vi "SimulationsLIA-Simulator.vi"() -> ()   [LabVIEW 2018]
uses:
  <vilib>/addons/Digital Filter Design/_Objects.llb/DFD Multirate Filter Specification (Design).ctl
  <vilib>/addons/Digital Filter Design/_Objects.llb/DFD Filter Ripple Specification (Design).ctl
  <vilib>/Analysis/4window.llb/windowTd.ctl
  <vilib>/addons/Digital Filter Design/Design.llb/DFD MRate Filter Design (Integer).vi
  <vilib>/addons/Digital Filter Design/Multirate.llb/DFD MRate Filtering (Array).vi
  <vilib>/measure/maspectr.llb/FFT Power Spectrum and PSD for 1 Chan (CDB).vi
  <vilib>/measure/maspectr.llb/FFT Power Spectrum and PSD for 1 Chan.vi
  <vilib>/measure/NI_MAPro.lvlib
  <vilib>/Analysis/NI_AALPro.lvlib
  <vilib>/addons/Digital Filter Design/NI_DigFilterLicensed.lvlib
  <vilib>/Analysis/NI_AALBase.lvlib
  <vilib>/addons/Digital Filter Design/Analysis.llb/DFD Plot Freq Response (Linear-Spaced).vi
panel:
  in  "Iterations":i32=10
  out "FFT Gain":dbl
  out "Audio Depth":dbl format="%#_p"
  in  "Resolution":dbl=19.0 format="%#_13g"
  in  "Sampling Rate":dbl=1.0 format="%#_p"
  in  "Number Samples":i32=10000
  out "Error Out":errorcluster
  in  "Error In":errorcluster
  in  "Stop":bool
  in  "Tab Control 3":enum32{"Signal", "Noise", "Decimated"}(tab)
  out "Noise vrms":dbl
  out "Noise (W|50ohms)":dbl
  out "k":dbl
  out "standard deviation":dbl format="%0.2p"
  out "mean":dbl format="%0.2p"
  in  "Tab Control 2":T1(tab)
  out "Waveform Graph 1":dbl[][](graph)
  out "Waveform Graph 3":cluster{"f0":dbl, "df":dbl, "magnitude":dbl[]}(graph)
  out "Waveform Graph 8":dbl[][](graph)
  out "Waveform Graph 7":cluster{"f0":dbl, "df":dbl, "magnitude":dbl[]}(graph)
  out "Waveform Graph 10":dbl[](graph)
  out "Waveform Graph 9":cluster{"f0":dbl, "df":dbl, "magnitude":dbl[]}(graph)
  out "Waveform Graph 12":dbl[](graph)
  out "Waveform Graph 11":cluster{"f0":dbl, "df":dbl, "magnitude":dbl[]}(graph)
  out "Waveform Graph 14":dbl[][](graph)
  out "Waveform Graph 13":cluster{"f0":dbl, "df":dbl, "magnitude":dbl[]}(graph)
  out "Waveform Graph 16":dbl[](graph)
  out "Waveform Graph 15":cluster{"f0":dbl, "df":dbl, "magnitude":dbl[]}(graph)
  in  "Tab Control 1":T2(tab)
  in  "Oscillator Frequency":dbl=-0.1 format="%#_p"
  in  "Oscillator Magnitude":dbl=1.0 format="%#_13g"
  in  "Signal Frequency":dbl=0.1 format="%#_p"
  in  "Signal Offset":cdb format="%#_13g"
  in  "Singal Amplitude":dbl=1.0 format="%#_13g"
  in  "Desired SNR (dB)":dbl format="%#_p"
  in  "freq specs [Hz]":T3={"fpass"=0.001, "fstop"=0.002}
  in  "ripple specs":T4={"passband"=0.1, "stopband"=70.0, "dB/linear? (T: dB)"=TRUE}
  in  "Decimation":i32=100
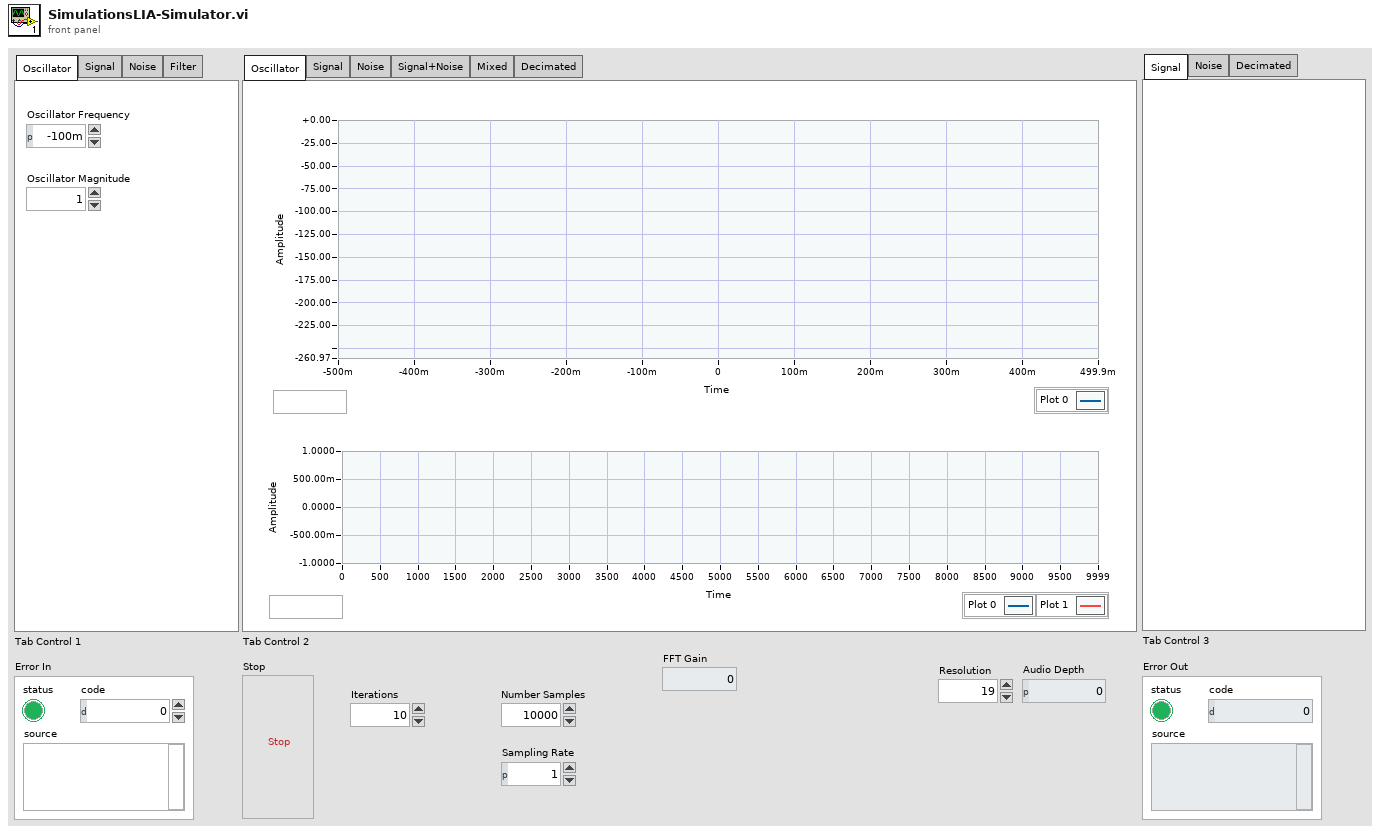
[diagram p1: front panel]
types:
  T1 = enum32{"Oscillator", "Signal", "Noise", "Signal+Noise", "Mixed", "Decimated"}
  T2 = enum32{"Oscillator", "Signal", "Noise", "Filter"}
  T3 = typedef "NI_DigFilterLicensed.lvlib/DFD Multirate Filter Specification (Design).ctl" = cluster{"fpass":dbl, "fstop":dbl}
  T4 = typedef "NI_DigFilterLicensed.lvlib/DFD Filter Ripple Specification (Design).ctl" = cluster{"passband":dbl, "stopband":dbl, "dB/linear? (T: dB)":bool}
  T5 = typedef "NI_DigFilterLicensed.lvlib/DFD Multirate Filter Obj.ctl" = cluster{"mMRate_Structure":enum16{"CIC", "FIR", "IIR", "Lattice"}, "mMRate_Mode":T6, "mMRate_Factor":i32, "mMRate_FIRParams":cluster{"mMRate_FIR_H":dbl[], "mMRate_FIR_IsNyquist?":bool, "mMRate_FIR_IsSymmetric?":bool}, "mMRate_CICParams":cluster{"mMRate_CIC_#Stage":i32, "mMRate_CIC_Lag":i32, "mMRate_CIC_Type":enum16{"Lowpass", "Highpass"}}, "mMRate_Order":i32, "mMRate_Version":string, "mMRate_Comments":string, "mMRate_RationalFactor":cluster{"mMRate_L":i32, "mMRate_M":i32}, "mMRate_Fs":dbl, "mMRate_Quantized?":bool, "mMRate_QFilterGain":dbl, "mMRate_CoefWl":i16, "mMRate_Scaling":cluster{"mMRate_ScaleByPowerOf2?":bool, "mMRate_ScaleType":T7}, "mMRate_InputWl":i16, "mMRate_OutputWl":i16, "mMRate_OutputMode":T8, "mMRate_MultMode":T9, "mMRate_BitPruning":bool, "mMRate_GainWl":i16, "mMRate_OutputFwl":i16, "mMRate_SumIwl":i16, "mMRate_InputIwl ":i16, "mMRate_SumWl":i16, "mMRate_CoefIwl":i16}
  T6 = typedef "NI_DigFilterLicensed.lvlib/DFD Multirate Mode.ctl" = i16
  T7 = typedef "NI_DigFilterLicensed.lvlib/DFD Coef Norm Type.ctl" = enum16{"No Norm", "Time Domain 1-Norm", "Time Domain 2-Norm", "Time Domain Inf-Norm"}
  T8 = typedef "NI_DigFilterLicensed.lvlib/DFD Round-off Mode.ctl" = enum16{"Nearest", "Truncation"}
  T9 = typedef "NI_DigFilterLicensed.lvlib/DFD FXP MRate Multiply Mode.ctl" = enum16{"Truncated", "Full"}
  T10 = cluster{"averaging mode":enum16{"No averaging", "Vector averaging", "RMS averaging", "Peak hold"}, "weighting mode":enum16{"Linear", "Exponential"}, "number of averages":u32}
  T11 = typedef "NI_AALPro.lvlib/windowTd.ctl" = u32
  T12 = typedef "NI_DigFilterLicensed.lvlib/DFD Filter Obj.ctl" = cluster{"mSRate_Fs":dbl, "mSRate_Version":string, "mSRate_Comments":string, "mSRate_OrgCoef":T13, "mSRate_CurCoef":T13, "mSRate_Quantized?":bool, "mSRate_QCoef":T13, "mSRate_QSettings":T15[], "mSRate_Order":i32, "mSRate_Scaling":cluster{"mSRate_ScaleByPowerOf2?":bool, "mSRate_ScaleType":T7}}
  T13 = typedef "NI_DigFilterLicensed.lvlib/DFD Filter Coef.ctl" = cluster{"type":T14, "gain":dbl, "coef a (k)":dbl[], "coef b (v)":dbl[]}
  T14 = typedef "NI_DigFilterLicensed.lvlib/DFD Filter Structure Type Selector.ctl" = enum16{"Undefined", "FIR Direct Form", "FIR Direct Form Transposed", "FIR Symmetric", "FIR Antisymmetric", "IIR Direct Form I", "IIR Direct Form I Transposed", "IIR Direct Form II", "IIR Direct Form II Transposed", "IIR Cascaded Second Order Sections Form I", "IIR Cascaded Second Order Sections Form I Transposed", "IIR Cascaded Second Order Sections Form II", "IIR Cascaded Second Order Sections Form II Transposed", "Lattice Allpass (basic sections)", "Lattice Allpass (one multiplier sections)", "Lattice Allpass (normalized sections)", "Lattice AR (basic sections)", "Lattice AR (one multiplier sections)", "Lattice AR (normalized sections)", "Lattice MA (minimum phase)", "Lattice MA (maximum phase)", "Lattice ARMA (basic sections)", "Lattice ARMA (one multiplier sections)", "Lattice ARMA (normalized sections)"}
  T15 = typedef "NI_DigFilterLicensed.lvlib/dfd_Internal Quantization Settings.ctl" = cluster{"source":T16, "wl":i16, "iwl":i16, "overflow mode":enum16{"Saturation", "Wrap"}, "rounding mode":enum16{"Nearest", "Truncation"}, "signed?":bool}
  T16 = typedef "NI_DigFilterLicensed.lvlib/dfd_Internal Quantization Srcs.ctl" = u16
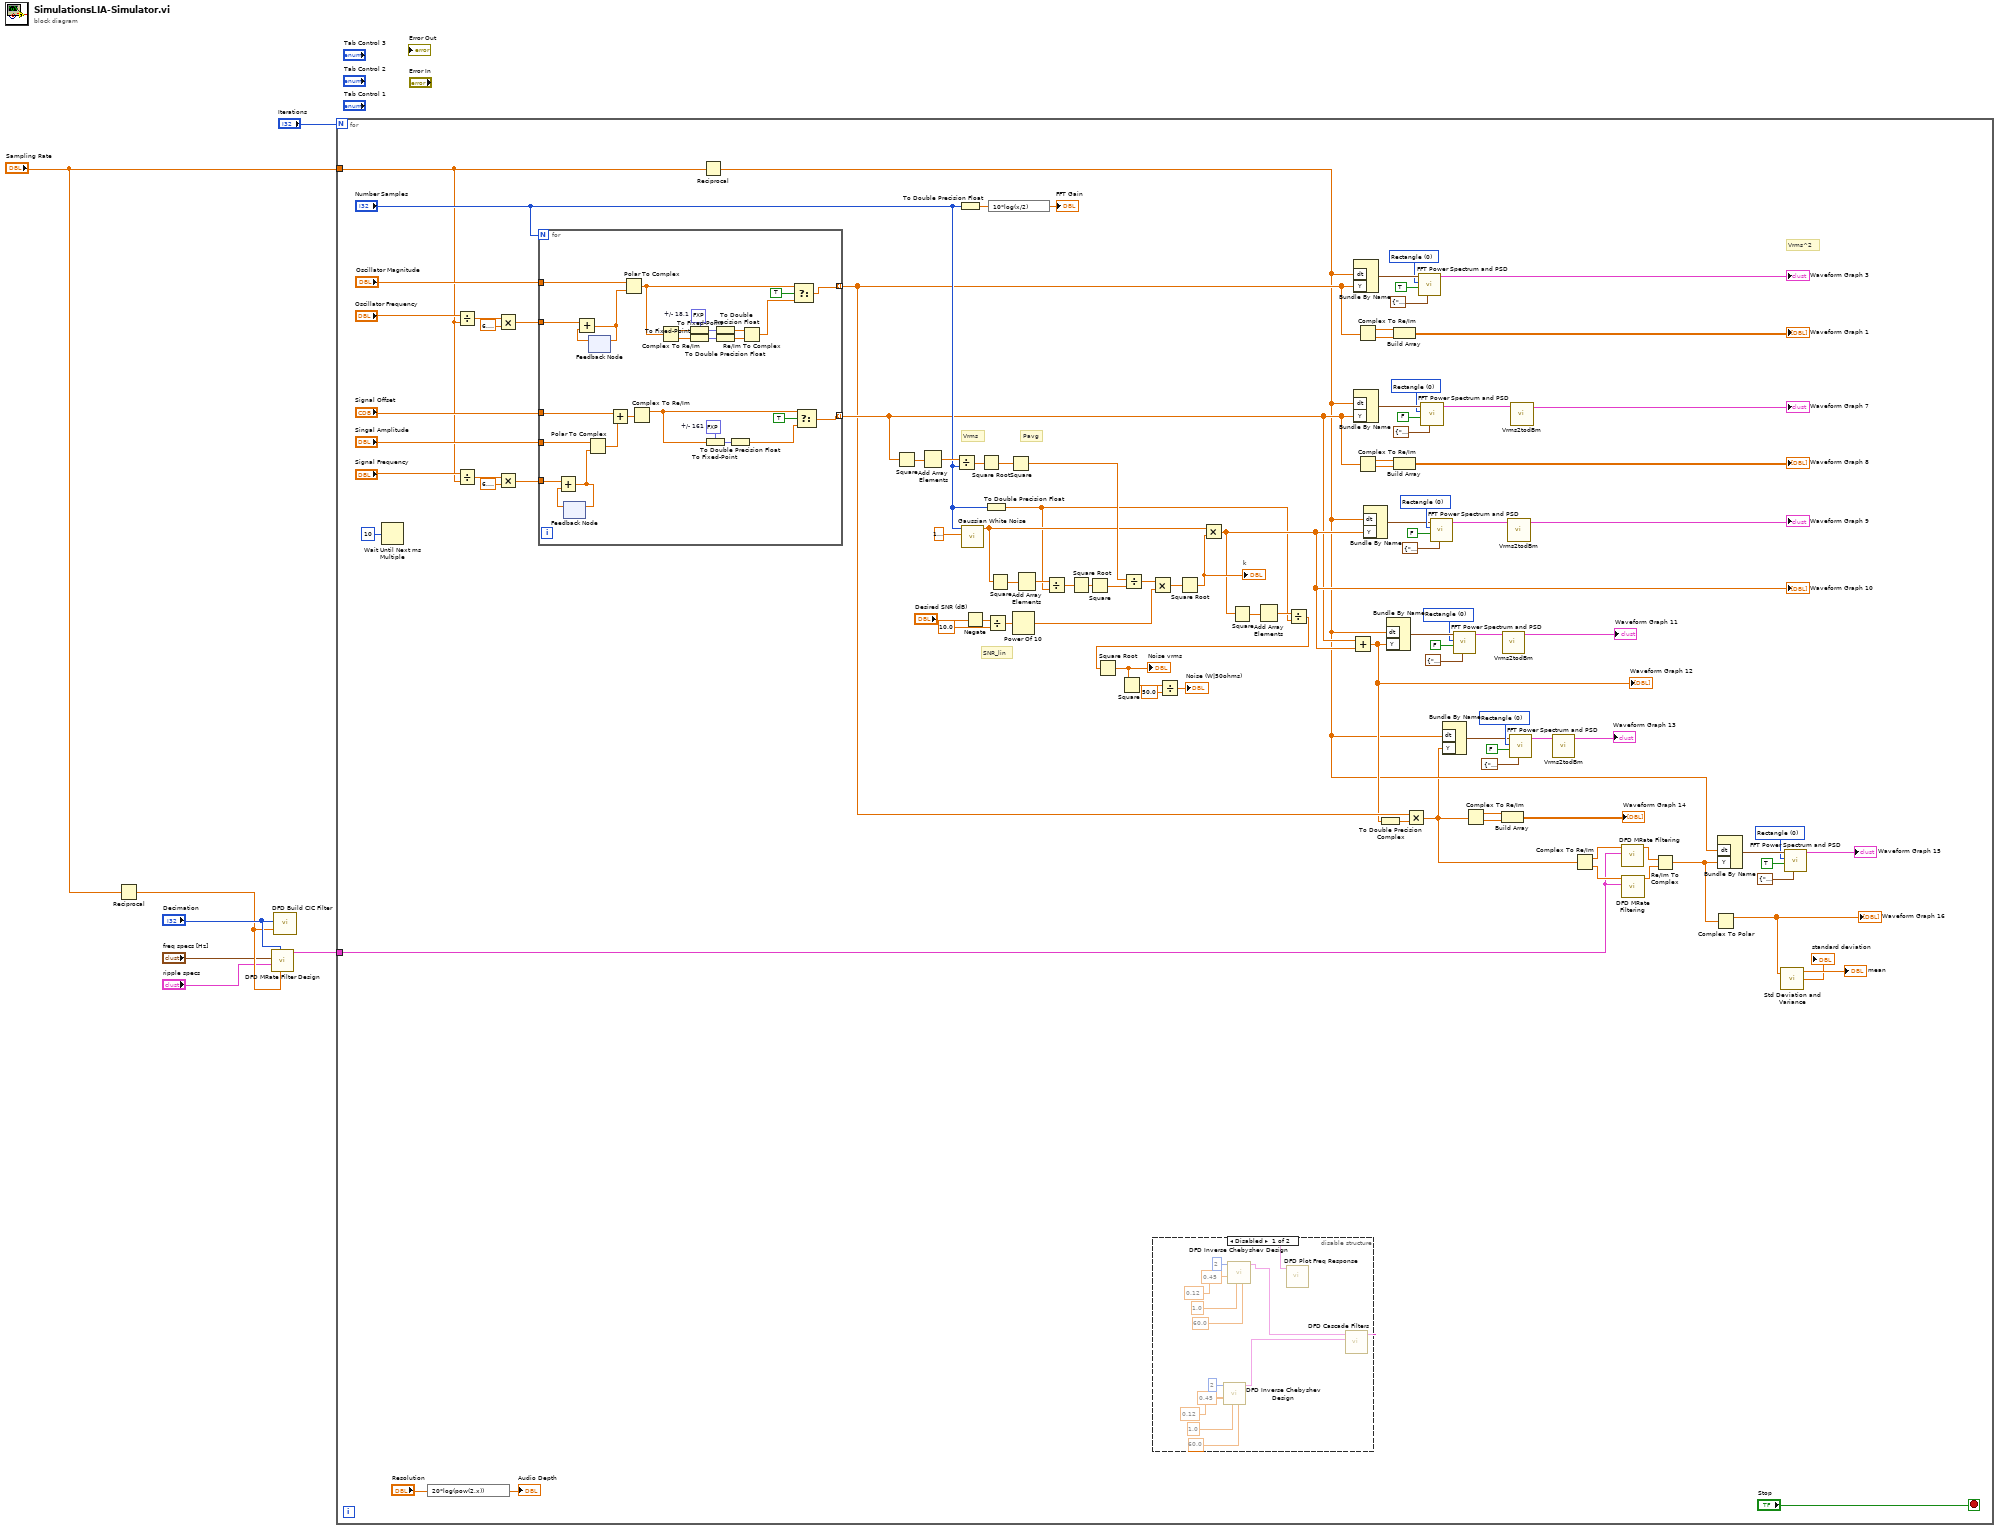
[diagram p0: block diagram]
diagram:
  n1 = Reciprocal(x="Sampling Rate") -> (1/x=w6:dbl)
  n2 = call-poly <vilib>:"DFD MRate Filter Design.vi"("fs in [Hz]"=w6, "factor"="Decimation", "ripple specs"="ripple specs", "freq specs [Hz]"="freq specs [Hz]") -> ("multirate filter out"=w2:T5)  [unwired: 6 in, 1 out]
  n3 = call <vilib>:"DFD Build CIC Filter.vi"("fs in [Hz]"=w6, "factor"="Decimation") -> ()  [unwired: 8 in, 2 out]
  n4 = for {
    N: "Iterations" -> [_]
    tunnel: "Sampling Rate" -> [w13]
    tunnel: w2 -> [w12]
    stop <- "Stop" stop-if-true
    w21 = T11 0 items=["Rectangle"=0, "Hanning"=1, "Hamming"=2, "Blackman-Harris"=3, "Exact Blackman"=4, "Blackman"=5, "Flat Top"=6, "4 Term B-Harris "=7, "7 Term B-Harris"=8, "Low Sidelobe"=9, "Blackman Nuttall"=11, "Triangle"=30, "Bartlett-Hanning"=31, "Bohman"=32, "Parzen"=33, "Welch"=34, "Kaiser"=60, "Dolph-Chebyshev"=61, "Gaussian"=62] ("window")
    w36 = T11 0 items=["Rectangle"=0, "Hanning"=1, "Hamming"=2, "Blackman-Harris"=3, "Exact Blackman"=4, "Blackman"=5, "Flat Top"=6, "4 Term B-Harris "=7, "7 Term B-Harris"=8, "Low Sidelobe"=9, "Blackman Nuttall"=11, "Triangle"=30, "Bartlett-Hanning"=31, "Bohman"=32, "Parzen"=33, "Welch"=34, "Kaiser"=60, "Dolph-Chebyshev"=61, "Gaussian"=62] ("window")
    w47 = T11 0 items=["Rectangle"=0, "Hanning"=1, "Hamming"=2, "Blackman-Harris"=3, "Exact Blackman"=4, "Blackman"=5, "Flat Top"=6, "4 Term B-Harris "=7, "7 Term B-Harris"=8, "Low Sidelobe"=9, "Blackman Nuttall"=11, "Triangle"=30, "Bartlett-Hanning"=31, "Bohman"=32, "Parzen"=33, "Welch"=34, "Kaiser"=60, "Dolph-Chebyshev"=61, "Gaussian"=62] ("window")
    w89 = T11 0 items=["Rectangle"=0, "Hanning"=1, "Hamming"=2, "Blackman-Harris"=3, "Exact Blackman"=4, "Blackman"=5, "Flat Top"=6, "4 Term B-Harris "=7, "7 Term B-Harris"=8, "Low Sidelobe"=9, "Blackman Nuttall"=11, "Triangle"=30, "Bartlett-Hanning"=31, "Bohman"=32, "Parzen"=33, "Welch"=34, "Kaiser"=60, "Dolph-Chebyshev"=61, "Gaussian"=62] ("window")
    w93 = T11 0 items=["Rectangle"=0, "Hanning"=1, "Hamming"=2, "Blackman-Harris"=3, "Exact Blackman"=4, "Blackman"=5, "Flat Top"=6, "4 Term B-Harris "=7, "7 Term B-Harris"=8, "Low Sidelobe"=9, "Blackman Nuttall"=11, "Triangle"=30, "Bartlett-Hanning"=31, "Bohman"=32, "Parzen"=33, "Welch"=34, "Kaiser"=60, "Dolph-Chebyshev"=61, "Gaussian"=62] ("window")
    w101 = T11 0 items=["Rectangle"=0, "Hanning"=1, "Hamming"=2, "Blackman-Harris"=3, "Exact Blackman"=4, "Blackman"=5, "Flat Top"=6, "4 Term B-Harris "=7, "7 Term B-Harris"=8, "Low Sidelobe"=9, "Blackman Nuttall"=11, "Triangle"=30, "Bartlett-Hanning"=31, "Bohman"=32, "Parzen"=33, "Welch"=34, "Kaiser"=60, "Dolph-Chebyshev"=61, "Gaussian"=62] ("window")
    # "SNR_lin"
    # "Pavg"
    # "Vrms"
    # "Vrms^2"
    n5 = Wait Until Next ms Multiple(millisecond multiple=u32 10) -> ()  [unwired: 1 out]
    n6 = expression code="20*log(pow(2,x))"("Resolution") -> (→"Audio Depth":dbl)
    n7 = Divide(x="Oscillator Frequency", y=w13) -> (x/y=w85:dbl)
    n8 = Divide(x="Signal Frequency", y=w13) -> (x/y=w111:dbl)
    n9 = Multiply(x=w85, y=6.283185307179586) -> (x*y=w82:dbl)
    n10 = Multiply(x=w111, y=6.283185307179586) -> (x*y=w110:dbl)
    n11 = for {
      N: "Number Samples" -> [_]
      tunnel: w110 -> [w150]
      tunnel: "Singal Amplitude" -> [w153]
      tunnel: "Signal Offset" -> [w152]
      tunnel: [w136] -> w38 mode=indexing
      tunnel: [w130] -> w40 mode=indexing
      tunnel: w82 -> [w141]
      tunnel: "Oscillator Magnitude" -> [w139]
      w131 = fxp<+/-,16,1> 0.0  # +/- 161
      w146 = fxp<+/-,18,1> 0.0  # +/- 18,1
      n12 = feedback #1() -> (w154:dbl)  [unwired: 1 in]
      n13 = Add(x=w150, y=w154) -> (x+y=w149:dbl)
      n14 = feedback-in #1(w149) -> ()
      n15 = Polar To Complex(1:w149, 2:w153) -> (0:w151:cdb)
      n16 = feedback #2() -> (w140:dbl)  [unwired: 1 in]
      n17 = Add(x=w141, y=w140) -> (x+y=w138:dbl)
      n18 = feedback-in #2(w138) -> ()
      n19 = Add(x=w152, y=w151) -> (x+y=w128:cdb)
      n20 = Polar To Complex(1:w138, 2:w139) -> (0:w137:cdb)
      n21 = Complex To Re/Im(x + iy=w128) -> (x=w127:dbl)  [unwired: 1 out]
      n22 = Complex To Re/Im(x + iy=w137) -> (x=w148:dbl, y=w147:dbl)
      n23 = To Fixed-Point(fixed-point type=w146, number=w148) -> (fixed-point=w145:fxp<+/-,18,1>)
      n24 = To Fixed-Point(fixed-point type=w146, number=w147) -> (fixed-point=w144:fxp<+/-,18,1>)
      n25 = To Fixed-Point(fixed-point type=w131, number=w127) -> (fixed-point=w132:fxp<+/-,16,1>)
      n26 = To Double Precision Float(number=w145) -> (double precision float=w143:dbl)
      n27 = To Double Precision Float(number=w144) -> (double precision float=w142:dbl)
      n28 = To Double Precision Float(number=w132) -> (double precision float=w129:dbl)
      n29 = Re/Im To Complex(1:w142, 2:w143) -> (0:w135:cdb)
      n30 = Select(t=w137, s=TRUE, f=w135) -> (s? t:f=w136:cdb)
      n31 = Select(t=w127, s=TRUE, f=w129) -> (s? t:f=w130:dbl)
    }
    n32 = Reciprocal(x=w13) -> (1/x=w20:dbl)
    n33 = Square(x=w40) -> (x^2=w80:dbl[])
    n34 = Add Array Elements(numeric array=w80) -> (sum=w79:dbl)
    n35 = Divide(x=w79, y="Number Samples") -> (x/y=w78:dbl)
    n36 = To Double Precision Float(number="Number Samples") -> (double precision float=w42:dbl)
    n37 = call <vilib>:"Gaussian White Noise.vi"("standard deviation"=1.0000000000000002, "samples"="Number Samples") -> ("Gaussian noise pattern"=w62:dbl[])  [unwired: 8 in, 1 out]
    n38 = Negate(x="Desired SNR (dB)") -> (-x=w65:dbl)
    n39 = Square Root(x=w78) -> (sqrt(x)=w77:dbl)
    n40 = To Double Precision Float(number="Number Samples") -> (double precision float=w29:dbl)
    n41 = Divide(x=w65, y=10.0) -> (x/y=w73:dbl)
    n42 = expression code="10*log(x/2)"(w42) -> (→"FFT Gain":dbl)
    n43 = Square(x=w62) -> (x^2=w69:dbl[])
    n44 = Square(x=w77) -> (x^2=w68:dbl)
    n45 = Power Of 10(x=w73) -> (10^x=w64:dbl)
    n46 = Add Array Elements(numeric array=w69) -> (sum=w70:dbl)
    n47 = Divide(x=w70, y=w29) -> (x/y=w71:dbl)
    n48 = Square Root(x=w71) -> (sqrt(x)=w72:dbl)
    n49 = Square(x=w72) -> (x^2=w67:dbl)
    n50 = Divide(x=w68, y=w67) -> (x/y=w66:dbl)
    n51 = Multiply(x=w66, y=w64) -> (x*y=w63:dbl)
    n52 = disable-structure shown="Disabled" {
      frame Disabled {
        n53 = call <vilib>:"DFD Inverse Chebyshev Design.vi"("stopband atten [dB]"=60.0, "fs [Hz]"=1.0, "low cutoff freq [Hz]"=0.12, "high cutoff freq [Hz]"=0.45, "order"=2) -> ("filter out"=w115:T12)  [unwired: 5 in, 1 out]
        n54 = call <vilib>:"DFD Inverse Chebyshev Design.vi"("stopband atten [dB]"=60.0, "fs [Hz]"=1.0, "low cutoff freq [Hz]"=0.12, "high cutoff freq [Hz]"=0.45, "order"=2) -> ("filter out"=w121:T12)  [unwired: 5 in, 1 out]
        n55 = call <vilib>:"DFD Cascade Filters.vi"("filter in 2"=w115, "filter in 1"=w121) -> ("filter out"=w114:T12)  [unwired: 8 in, 1 out]
        n56 = call-poly <vilib>:"DFD Plot Freq Response.vi"("filter in"=w114) -> ()  [unwired: 7 in, 4 out]
      }
      frame Enabled {
      }
    }
    n57 = Square Root(x=w63) -> (sqrt(x)=w61:dbl)
    "k" <- w61
    n58 = Multiply(x=w62, y=w61) -> (x*y=w46:dbl[])
    "Waveform Graph 10" <- w46
    n59 = Square(x=w46) -> (x^2=w59:dbl[])
    n60 = Add Array Elements(numeric array=w59) -> (sum=w58:dbl)
    n61 = Divide(x=w58, y=w29) -> (x/y=w57:dbl)
    n62 = Square Root(x=w57) -> (sqrt(x)=w56:dbl)
    "Noise vrms" <- w56
    n63 = Square(x=w56) -> (x^2=w55:dbl)
    n64 = Divide(x=w55, y=50.0) -> (x/y=→"Noise (W|50ohms)":dbl)
    n65 = Add(x=w40, y=w46) -> (x+y=w37:dbl[])
    "Waveform Graph 12" <- w37
    n66 = Bundle By Name("dt"=w20, "Y"=w38) -> (w104:waveform(cdb))  [unwired: 1 in]
    n67 = Bundle By Name("dt"=w20, "Y"=w40) -> (w96:waveform(dbl))  [unwired: 1 in]
    n68 = Complex To Re/Im(x + iy=w38) -> (x=w99:dbl[], y=w98:dbl[])
    n69 = Complex To Re/Im(x + iy=w40) -> (x=w92:dbl[], y=w91:dbl[])
    n70 = Bundle By Name("dt"=w20, "Y"=w46) -> (w86:waveform(dbl))  [unwired: 1 in]
    n71 = To Double Precision Complex(1:w37) -> (0:w17:cdb[])
    n72 = Bundle By Name("dt"=w20, "Y"=w37) -> (w50:waveform(dbl))  [unwired: 1 in]
    n73 = Build Array(w99, w98) -> (→"Waveform Graph 1":dbl[][])
    n74 = Build Array(w92, w91) -> (→"Waveform Graph 8":dbl[][])
    n75 = Multiply(x=w38, y=w17) -> (x*y=w16:cdb[])
    n76 = call-poly <vilib>:"FFT Power Spectrum and PSD.vi"("averaging parameters"=T10 {"averaging mode"=enum."No averaging", "weighting mode"=enum."Exponential", "number of averages"=10}, "dB On (F)"=TRUE, "window"=w101, "time signal"=w104) -> ("Power Spectrum / PSD"=→"Waveform Graph 3":cluster{"f0":dbl, "df":dbl, "magnitude":dbl[]})  [unwired: 4 in, 3 out]
    n77 = call-poly <vilib>:"FFT Power Spectrum and PSD.vi"("averaging parameters"=T10 {"averaging mode"=enum."RMS averaging", "weighting mode"=enum."Exponential", "number of averages"=10}, "dB On (F)"=FALSE, "window"=w93, "time signal"=w96) -> ("Power Spectrum / PSD"=w39:cluster{"f0":dbl, "df":dbl, "magnitude":dbl[]})  [unwired: 4 in, 3 out]
    n78 = call-poly <vilib>:"FFT Power Spectrum and PSD.vi"("averaging parameters"=T10 {"averaging mode"=enum."RMS averaging", "weighting mode"=enum."Exponential", "number of averages"=10}, "dB On (F)"=FALSE, "window"=w89, "time signal"=w86) -> ("Power Spectrum / PSD"=w44:cluster{"f0":dbl, "df":dbl, "magnitude":dbl[]})  [unwired: 4 in, 3 out]
    n79 = Bundle By Name("dt"=w20, "Y"=w16) -> (w33:waveform(cdb))  [unwired: 1 in]
    n80 = call-poly <vilib>:"FFT Power Spectrum and PSD.vi"("averaging parameters"=T10 {"averaging mode"=enum."RMS averaging", "weighting mode"=enum."Exponential", "number of averages"=10}, "dB On (F)"=FALSE, "window"=w47, "time signal"=w50) -> ("Power Spectrum / PSD"=w51:cluster{"f0":dbl, "df":dbl, "magnitude":dbl[]})  [unwired: 4 in, 3 out]
    n81 = Complex To Re/Im(x + iy=w16) -> (x=w31:dbl[], y=w32:dbl[])
    n82 = Build Array(w31, w32) -> (→"Waveform Graph 14":dbl[][])
    n83 = call "Vrms2todBm.vi"("Power Spectrum / PSD in"=w51) -> ("Power Spectrum / PSD out"=→"Waveform Graph 11":cluster{"f0":dbl, "df":dbl, "magnitude":dbl[]})  [unwired: 10 in]
    n84 = call "Vrms2todBm.vi"("Power Spectrum / PSD in"=w44) -> ("Power Spectrum / PSD out"=→"Waveform Graph 9":cluster{"f0":dbl, "df":dbl, "magnitude":dbl[]})  [unwired: 10 in]
    n85 = call-poly <vilib>:"FFT Power Spectrum and PSD.vi"("averaging parameters"=T10 {"averaging mode"=enum."RMS averaging", "weighting mode"=enum."Exponential", "number of averages"=10}, "dB On (F)"=FALSE, "window"=w36, "time signal"=w33) -> ("Power Spectrum / PSD"=w15:cluster{"f0":dbl, "df":dbl, "magnitude":dbl[]})  [unwired: 4 in, 3 out]
    n86 = call "Vrms2todBm.vi"("Power Spectrum / PSD in"=w39) -> ("Power Spectrum / PSD out"=→"Waveform Graph 7":cluster{"f0":dbl, "df":dbl, "magnitude":dbl[]})  [unwired: 10 in]
    n87 = call "Vrms2todBm.vi"("Power Spectrum / PSD in"=w15) -> ("Power Spectrum / PSD out"=→"Waveform Graph 13":cluster{"f0":dbl, "df":dbl, "magnitude":dbl[]})  [unwired: 10 in]
    n88 = Complex To Re/Im(x + iy=w16) -> (x=w28:dbl[], y=w27:dbl[])
    n89 = call-poly <vilib>:"DFD MRate Filtering.vi"("multirate filter"=w12, "signal in"=w28) -> ("signal out"=w25:dbl[])  [unwired: 8 in, 1 out]
    n90 = call-poly <vilib>:"DFD MRate Filtering.vi"("multirate filter"=w12, "signal in"=w27) -> ("signal out"=w26:dbl[])  [unwired: 8 in, 1 out]
    n91 = Re/Im To Complex(1:w26, 2:w25) -> (0:w18:cdb[])
    n92 = Complex To Polar(r * e^(i*theta)=w18) -> (r=w10:dbl[])  [unwired: 1 out]
    "Waveform Graph 16" <- w10
    n93 = Bundle By Name("dt"=w20, "Y"=w18) -> (w24:waveform(cdb))  [unwired: 1 in]
    n94 = call <vilib>:"Std Deviation and Variance.vi"("X"=w10) -> ("mean"=→"mean":dbl, "standard deviation"=→"standard deviation":dbl)  [unwired: 1 in, 1 out]
    n95 = call-poly <vilib>:"FFT Power Spectrum and PSD.vi"("averaging parameters"=T10 {"averaging mode"=enum."RMS averaging", "weighting mode"=enum."Exponential", "number of averages"=10}, "dB On (F)"=TRUE, "window"=w21, "time signal"=w24) -> ("Power Spectrum / PSD"=→"Waveform Graph 15":cluster{"f0":dbl, "df":dbl, "magnitude":dbl[]})  [unwired: 4 in, 3 out]
  }
